vi "PAQmem_ReadArray.vi"(8 "error in (no error)":errorcluster, 10 "ChunkDefinition":T2, 11 "PAQ-memory in":refnum<class "PAQ-memory.lvclass">) -> (0 "error out":errorcluster, 2 "GraphData":T1, 3 "PAQ-memory out":refnum<class "PAQ-memory.lvclass">)   [LabVIEW 2014, in "PAQ-memory.lvclass"]
doc: "For One TAG get an Array of data"
uses:
  PAQ-memory.lvclass
  PAQ-memory.lvclass/PAQ-memory.ctl
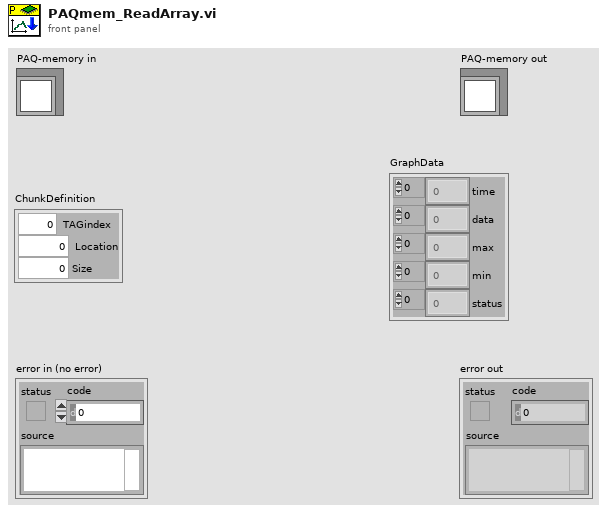
[diagram p1: front panel]
types:
  T1 = cluster{"time":dbl[], "data":dbl[], "max":dbl[], "min":dbl[], "status":u32[]}
  T2 = cluster{"TAGindex":i32, "Location":i32, "Size":i32}
  T3 = cluster{"source":refnum<data-value>, "status":refnum<data-value>, "data":refnum<data-value>, "max":refnum<data-value>, "min":refnum<data-value>}[]
  T4 = cluster{"source":refnum<data-value>, "status":refnum<data-value>, "data":refnum<data-value>, "max":refnum<data-value>, "min":refnum<data-value>}
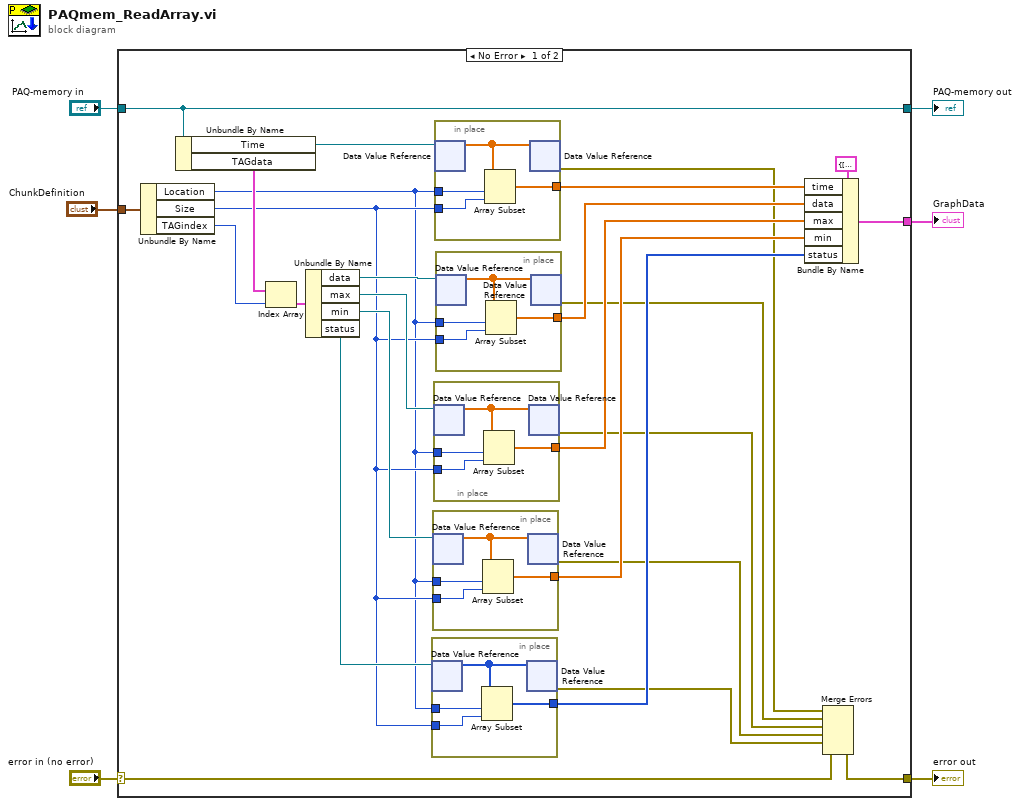
[diagram p0: block diagram]
diagram:
  n1 = case shown="No Error" "error in (no error)" {
    selector: "error in (no error)" -> [w13 w54]
    tunnel: [w7 w54] -> w5
    tunnel: [w31 w53] -> w3
    tunnel: "PAQ-memory in" -> [w31 w53]
    tunnel: "ChunkDefinition" -> [w32 _]
    tunnel: [w28 _] -> w1
    frame No Error {
      n2 = Unbundle By Name(w32) -> ("Location"=w14:i32, "Size"=w19:i32, "TAGindex"=w25:i32)
      n3 = Unbundle By Name(w31) -> ("Time"=w30:refnum<data-value>, "TAGdata"=w26:T3)
      n4 = Index Array(array=w26, index=w25) -> (element=w24:T4)
      n5 = Unbundle By Name(w24) -> ("data"=w23:refnum<data-value>, "max"=w22:refnum<data-value>, "min"=w21:refnum<data-value>, "status"=w20:refnum<data-value>)
      n6 = in-place {
        in-place-border: w14 -> [w35]
        in-place-border: w19 -> [w34]
        in-place-border: [w33] -> w15
        n7 = in-place-dvr #1(w20) -> (w36:u32[])  [unwired: 1 out]
        n8 = Array Subset(array=w36, index=w35, length=w34) -> (w33:u32[])
        n9 = in-place-dvr #1(w36) -> (w12:errorcluster)  [unwired: 1 out]
      }
      n10 = in-place {
        in-place-border: w14 -> [w39]
        in-place-border: w19 -> [w38]
        in-place-border: [w37] -> w16
        n11 = in-place-dvr #2(w21) -> (w40:dbl[])  [unwired: 1 out]
        n12 = Array Subset(array=w40, index=w39, length=w38) -> (w37:dbl[])
        n13 = in-place-dvr #2(w40) -> (w11:errorcluster)  [unwired: 1 out]
      }
      n14 = in-place {
        in-place-border: w14 -> [w43]
        in-place-border: w19 -> [w42]
        in-place-border: [w41] -> w17
        n15 = in-place-dvr #3(w22) -> (w44:dbl[])  [unwired: 1 out]
        n16 = Array Subset(array=w44, index=w43, length=w42) -> (w41:dbl[])
        n17 = in-place-dvr #3(w44) -> (w10:errorcluster)  [unwired: 1 out]
      }
      n18 = in-place {
        in-place-border: w14 -> [w51]
        in-place-border: w19 -> [w50]
        in-place-border: [w49] -> w27
        n19 = in-place-dvr #4(w30) -> (w52:dbl[])  [unwired: 1 out]
        n20 = Array Subset(array=w52, index=w51, length=w50) -> (w49:dbl[])
        n21 = in-place-dvr #4(w52) -> (w8:errorcluster)  [unwired: 1 out]
      }
      n22 = in-place {
        in-place-border: w14 -> [w47]
        in-place-border: w19 -> [w46]
        in-place-border: [w45] -> w18
        n23 = in-place-dvr #5(w23) -> (w48:dbl[])  [unwired: 1 out]
        n24 = Array Subset(array=w48, index=w47, length=w46) -> (w45:dbl[])
        n25 = in-place-dvr #5(w48) -> (w9:errorcluster)  [unwired: 1 out]
      }
      n26 = Bundle By Name(cluster=T1 {"time"=[], "data"=[], "max"=[], "min"=[], "status"=[]} ("GraphData"), "time"=w27, "data"=w18, "max"=w17, "min"=w16, "status"=w15) -> (w28:T1)
      n27 = Merge Errors(w8, w9, w10, w11, w12, w13) -> (w7:errorcluster)
    }
    frame Error {
    }
  }
  "error out" <- w5
  "PAQ-memory out" <- w3
  "GraphData" <- w1
